vi "3_МПА.vi"(11 "Уставка давления":dbl(slide)=0.02 min=0.02 max=2.0 step=0.001 scale=0.0..3.0) -> (3 "mka":u16(slide)=4001 scale=4000.0..20000.0)   [LabVIEW 2018]
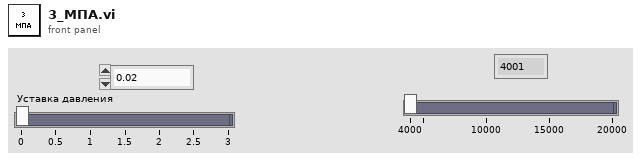
[diagram p1: front panel]
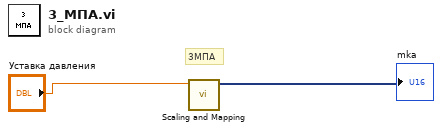
[diagram p0: block diagram]
diagram:
  # "3МПА"
  n1 = call "Scaling and Mapping"("Signals"="Уставка давления") -> ("Scaled Signals"=→"mka":dynamicdata)  [unwired: 9 in, 1 out]
